vi "Keyboard-Demo.vi"() -> ()   [LabVIEW 2016]
panel:
  in  "Windows System Language":enum16{"English", "German"}(ring)
  in  "Filename":string="c:\\test.txt"
  in  "Message to send":string="This VI demonstrates the operation of the Keyboard-Routines.\nIt opens Notepad, writes this text into it and saves it under the filename given below.\nPlease select your Windows System Language first, as the Notepad shortcuts depend on the language.\n\nIf you add a new Windows Language Version to this VI, please mail it to me so other LVers can profit. \n\nIf you're interested in new versions, please send me an email to eyfrigd@sick.de.\n\nYou may freely distribute these keyboard handling VIs, as long as you include all the files.\n\nGood luck\nDirk"
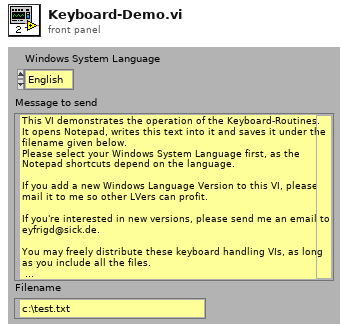
[diagram p1: front panel]
types:
  T1 = enum16{"Mouse Left", "Mouse Right", "Break", "Mouse Middle", "Backspace", "Tabulator", "FormFeed", "Return", "Shift", "Control", "Alternate", "Pause", "CapsLock", "Escape", "Space", "Page Up", "Page Down", "End", "Home", "Left", "Up", "Right", "Down", "Select", "Print", "Execute", "Snapshot", "Insert", "Delete", "Help", "0", "1", "2", "3", "4", "5", "6", "7", "8", "9", "A", "B", "C", "D", "E", "F", "G", "H", "I", "J", "K", "L", "M", "N", "O", "P", "Q", "R", "S", "T", "U", "V", "W", "X", "Y", "Z", "Win Left", "Win Right", "Context Menu", "Num 0", "Num 1", "Num 2", "Num 3", "Num 4", "Num 5", "Num 6", "Num 7", "Num 8", "Num 9", "Multiply", "Add", "Separator", "Subtract", "Decimal", "Divide", "F1", "F2", "F3", "F4", "F5", "F6", "F7", "F8", "F9", "F10", "F11", "F12", "F13", "F14", "F15", "F16", "F17", "F18", "F19", "F20", "F21", "F22", "F23", "F24", "NumLock", "Scroll", "Shift Left", "Shift Right", "Control Left", "Control Right", "Alternate Left", "Alternate Right", "Attn", "CrSel", "ExSel", "ErEOF", "Play", "Zoom", "Noname", "PA1", "OEM Clear", "Germany <", "Germany ^", "Germany ß", "Germany ´", "Germany ü", "Germany +", "Germany ö", "Germany ä", "Germany #", "Germany ,", "Germany .", "Germany -"}
  T2 = enum16{"NO", "SHIFT", "CTRL", "ALT", "SHIFT + CTRL", "SHIFT + ALT", "CTRL + ALT", "SHIFT + CTRL + ALT"}
  T3 = typedef "WindowHandle" = refnum<k1>
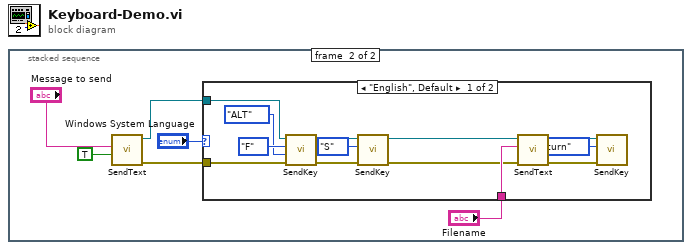
[diagram p0: block diagram]
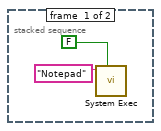
[diagram p2: hidden frame]
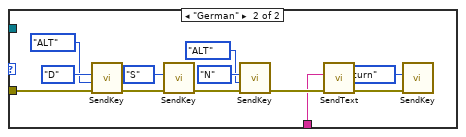
[diagram p3: hidden frame]
diagram:
  n1 = stacked-sequence {
    frame #0 {
      n2 = call <vilib>:"System Exec.vi"("wait until completion? (T)"=FALSE, "command line"="Notepad" ("command to execute")) -> ()  [unwired: 6 in, 4 out]
    }
    frame #1 {
      n3 = call "SendText.vi"("Replace LF"=TRUE, "Text"="Message to send") -> ("error out"=w7:errorcluster, "Previous WindowHandle"=w3:T3)  [unwired: 4 in]
      n4 = case shown="\"English\", Default" "Windows System Language" {
        tunnel: w7 -> [w21 w33]
        tunnel: "Filename" -> [w14 w22]
        tunnel: w3 -> [w9 _]
        frame "English", Default {
          n5 = call "SendKey.vi"("error in (no error)"=w21, "ShiftState"=T2."ALT", "Virtual Key"=T1."F", "WindowHandle"=w9) -> ("error out"=w19:errorcluster, "Previous WindowHandle"=w10:T3)  [unwired: 2 in]
          n6 = call "SendKey.vi"("error in (no error)"=w19, "Virtual Key"=T1."S", "WindowHandle"=w10) -> ("error out"=w13:errorcluster, "Previous WindowHandle"=w12:T3)  [unwired: 3 in]
          n7 = call "SendText.vi"("error in (no error)"=w13, "Text"=w14, "WindowHandle"=w12) -> ("error out"=w15:errorcluster, "Previous WindowHandle"=w11:T3)  [unwired: 3 in]
          n8 = call "SendKey.vi"("error in (no error)"=w15, "Virtual Key"=T1."Return", "WindowHandle"=w11) -> ()  [unwired: 3 in, 2 out]
        }
        frame "German" {
          n9 = call "SendKey.vi"("error in (no error)"=w33, "ShiftState"=T2."ALT", "Virtual Key"=T1."D") -> ("error out"=w31:errorcluster)  [unwired: 3 in, 1 out]
          n10 = call "SendKey.vi"("error in (no error)"=w31, "Virtual Key"=T1."S") -> ("error out"=w27:errorcluster)  [unwired: 4 in, 1 out]
          n11 = call "SendKey.vi"("error in (no error)"=w27, "ShiftState"=T2."ALT", "Virtual Key"=T1."N") -> ("error out"=w25:errorcluster)  [unwired: 3 in, 1 out]
          n12 = call "SendText.vi"("error in (no error)"=w25, "Text"=w22) -> ("error out"=w23:errorcluster)  [unwired: 4 in, 1 out]
          n13 = call "SendKey.vi"("error in (no error)"=w23, "Virtual Key"=T1."Return") -> ()  [unwired: 4 in, 2 out]
        }
      }
    }
  }
